vi "setConvertControl.vi"(8 "error in (no error)":errorcluster, 9 "convert_control":T2={"sharpen"=TRUE, "adaptive_sharpen"=TRUE, "flip_vertical"=FALSE, "auto_minmax"=TRUE, "add_conv_flags"=0, "min_limit"=20000, "max_limit"=1, "gamma"=0.0, "contrast"=0, "pco_debayer_algorithm"=FALSE, "color_temperature"=0, "color_saturation"=0, "color_vibrance"=0, "color_tint"=0, "lut_file"=path ""} {"max_limit" format="%#_6f"}, 10 "data_format":T1(ring)=enum."Mono16", 11 "Camera in":refnum<class "Camera.lvclass">) -> (0 "error out":errorcluster, 3 "Camera out":refnum<class "Camera.lvclass">)   [LabVIEW 2019, in "Camera.lvclass"]
doc: "Sets the paramerters for converting raw image data to other image formats."
uses:
  Camera.lvclass
  Camera.lvclass/Camera.ctl
  pco.convert/Convert.lvlib
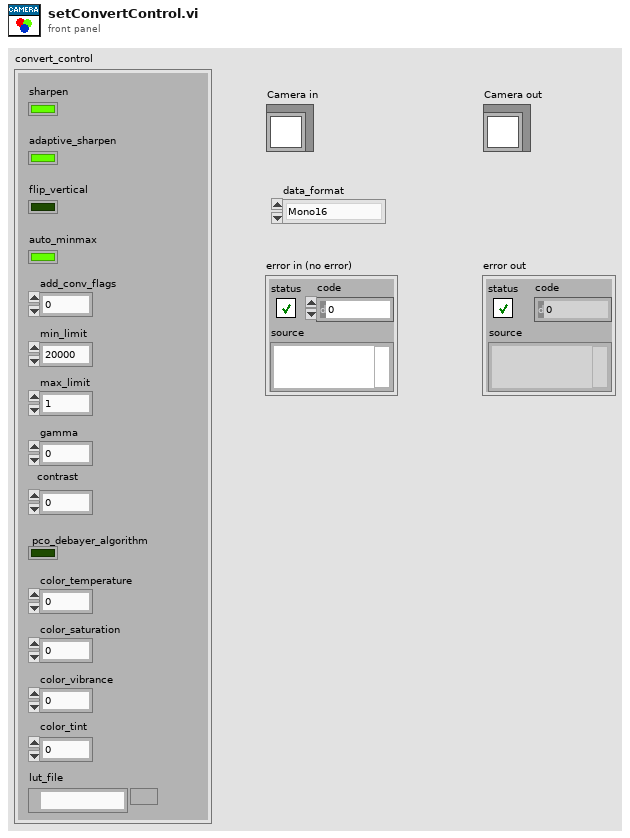
[diagram p1: front panel]
types:
  T1 = enum16{"Undefined", "Mono8", "Mono16", "BGRA8", "RGBA8", "BGRA16", "RGBA16", "CompressedMono8"}
  T2 = cluster{"sharpen":bool, "adaptive_sharpen":bool, "flip_vertical":bool, "auto_minmax":bool, "add_conv_flags":u32, "min_limit":u16, "max_limit":u16, "gamma":dbl, "contrast":i32, "pco_debayer_algorithm":bool, "color_temperature":i32, "color_saturation":i32, "color_vibrance":i32, "color_tint":i32, "lut_file":path}
  T3 = map{enum16{"Undefined", "Mono8", "Mono16", "BGRA8", "RGBA8", "BGRA16", "RGBA16", "CompressedMono8"}, cluster{"sharpen":bool, "adaptive_sharpen":bool, "flip_vertical":bool, "auto_minmax":bool, "add_conv_flags":u32, "min_limit":u16, "max_limit":u16, "gamma":dbl, "contrast":i32, "pco_debayer_algorithm":bool, "color_temperature":i32, "color_saturation":i32, "color_vibrance":i32, "color_tint":i32, "lut_file":path}}
  T4 = map{enum16{"Undefined", "Mono8", "Mono16", "BGRA8", "RGBA8", "BGRA16", "RGBA16", "CompressedMono8"}, u64}
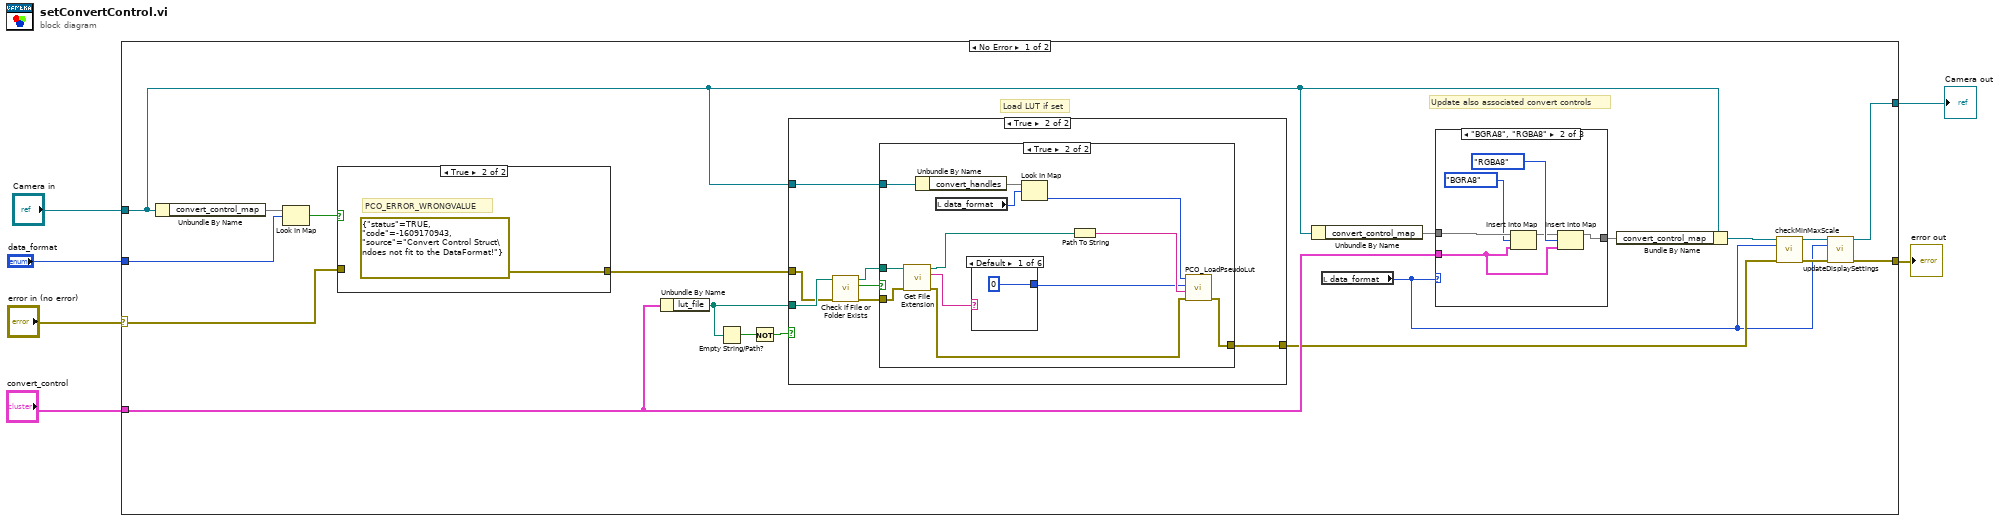
[diagram p0: block diagram]
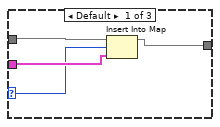
[diagram p2: hidden frame]
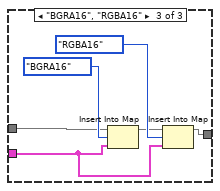
[diagram p3: hidden frame]
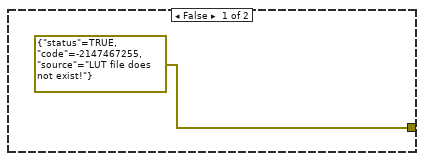
[diagram p5: hidden frame]
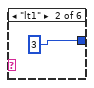
[diagram p6: hidden frame]
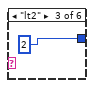
[diagram p7: hidden frame]
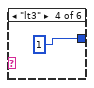
[diagram p8: hidden frame]
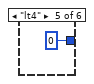
[diagram p9: hidden frame]
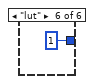
[diagram p10: hidden frame]
diagram:
  n1 = case shown="No Error" "error in (no error)" {
    selector: "error in (no error)" -> [w22 w72]
    tunnel: [w14 w72] -> w5
    tunnel: [w15 w71] -> w3
    tunnel: "Camera in" -> [w16 w71]
    tunnel: "convert_control" -> [w13 _]
    tunnel: "data_format" -> [w24 _]
    frame No Error {
      # "Update also associated convert controls"
      # "Load LUT if set"
      n2 = Unbundle By Name(w16) -> ("convert_control_map"=w25:T3)
      n3 = Look In Map(map=w25, key=w24) -> (key not found?=w23:bool)  [unwired: 1 in, 1 out]
      n4 = case shown="True" w23 {
        tunnel: w22 -> [w69 _]
        tunnel: [w69 errorcluster {"status"=TRUE, "code"=-1609170943, "source"="Convert Control Struct\ndoes not fit to the DataFormat!"} ("error IO")] -> w19
        frame False {
        }
        frame True {
          # "PCO_ERROR_WRONGVALUE"
        }
      }
      n5 = Unbundle By Name(w13) -> ("lut_file"=w18:path)
      n6 = Empty String/Path?(string/path=w18) -> (empty?=w21:bool)
      n7 = Not(x=w21) -> (.not. x?=w20:bool)
      n8 = case shown="True" w20 {
        tunnel: w19 -> [w42 w48]
        tunnel: w18 -> [_ w49]
        tunnel: w16 -> [_ w43]
        tunnel: [w42 w45] -> w9
        frame False {
        }
        frame True {
          n9 = call <vilib>:"Check if File or Folder Exists.vi"("error in (no error)"=w48, "path"=w49) -> ("error out"=w46:errorcluster, "file or folder exists?"=w47:bool, "dup path"=w44:path)  [unwired: 7 in]
          n10 = case shown="True" w47 {
            tunnel: w46 -> [_ w55]
            tunnel: [errorcluster {"status"=TRUE, "code"=-2147467255, "source"="LUT file does not exist!"} ("error IO") w53] -> w45
            tunnel: w44 -> [_ w59]
            tunnel: w43 -> [_ w62]
            frame False {
            }
            frame True {
              n11 = call <vilib>:"Get File Extension.vi"("error in (no error)"=w55, "file"=w59) -> ("error out"=w54:errorcluster, "lowercase file extension"=w52:string, "dup file"=w58:path)  [unwired: 5 in, 2 out]
              n12 = Unbundle By Name(w62) -> ("convert_handles"=w60:T4)
              n13 = local read "data_format"() -> (w61:T1)
              n14 = case shown="Default" w52 {
                tunnel: [0 ("format") 3 ("format") 2 ("format") 1 ("format") 0 ("format") 1 ("format")] -> w51
                frame Default {
                }
                frame "lt1" {
                }
                frame "lt2" {
                }
                frame "lt3" {
                }
                frame "lt4" {
                }
                frame "lut" {
                }
              }
              n15 = Look In Map(map=w60, key=w61) -> (value=w56:u64)  [unwired: 1 in, 1 out]
              n16 = Path To String(path=w58) -> (string=w57:string)
              n17 = call "PCO_LoadPseudoLut.vi"("error in (no error)"=w54, "filename"=w57, "format"=w51, "ph"=w56) -> ("error out"=w53:errorcluster)  [unwired: 5 in, 2 out]
            }
          }
        }
      }
      n18 = Unbundle By Name(w16) -> ("convert_control_map"=w17:T3)
      n19 = local read "data_format"() -> (w7:T1)
      n20 = case shown="\"BGRA8\", \"RGBA8\"" w7 {
        selector: w7 -> [w27 _ _]
        tunnel: w17 -> [w28 w35 w37]
        tunnel: w13 -> [w29 w33 w36]
        tunnel: [w26 w30 w38] -> w12
        frame Default {
          n21 = Insert Into Map(map in=w28, key=w27, value=w29) -> (map out=w26:T3)  [unwired: 2 out]
        }
        frame "BGRA8", "RGBA8" {
          n22 = Insert Into Map(map in=w35, key=T1."BGRA8" ("data_format"), value=w33) -> (map out=w31:T3)  [unwired: 2 out]
          n23 = Insert Into Map(map in=w31, key=T1."RGBA8" ("data_format"), value=w33) -> (map out=w30:T3)  [unwired: 2 out]
        }
        frame "BGRA16", "RGBA16" {
          n24 = Insert Into Map(map in=w37, key=T1."BGRA16" ("data_format"), value=w36) -> (map out=w39:T3)  [unwired: 2 out]
          n25 = Insert Into Map(map in=w39, key=T1."RGBA16" ("data_format"), value=w36) -> (map out=w38:T3)  [unwired: 2 out]
        }
      }
      n26 = Bundle By Name(cluster=w16, "convert_control_map"=w12) -> (w8:refnum<class "Camera.lvclass">)
      n27 = call-dynamic "checkMinMaxScale.vi"("Camera in"=w8, "data_format"=w7, "error in (no error)"=w9) -> ("Camera out"=w11:refnum<class "Camera.lvclass">, "error out"=w10:errorcluster)  [unwired: 10 in, 1 out]
      n28 = call-dynamic "updateDisplaySettings.vi"("Camera in"=w11, "data_format"=w7, "error in (no error)"=w10) -> ("Camera out"=w15:refnum<class "Camera.lvclass">, "error out"=w14:errorcluster)  [unwired: 11 in]
    }
    frame Error {
    }
  }
  "error out" <- w5
  "Camera out" <- w3
